vi "sensitivity.vi"(9 "x":dbl, 11 "sensitivity":dbl) -> (3 "scaled value":dbl)   [LabVIEW 2018]
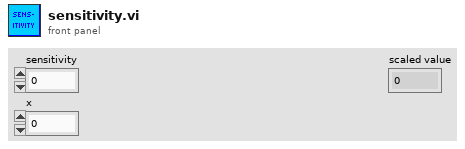
[diagram p1: front panel]
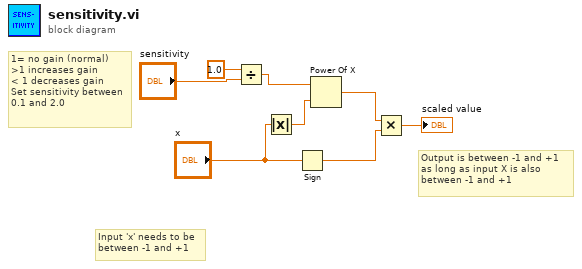
[diagram p0: block diagram]
diagram:
  # "Input 'x' needs to be\nbetween -1 and +1"
  # "Output is between -1 and +1\nas long as input X is also\nbetween -1 and +1"
  # "1= no gain (normal)\n>1 increases gain\n< 1 decreases gain\nSet sensitivity between\n0.1 and 2.0"
  n1 = Divide(x=1.0, y="sensitivity") -> (x/y=w8:dbl)
  n2 = Absolute Value(x="x") -> (abs(x)=w5:dbl)
  n3 = Sign(1:"x") -> (0:w2:dbl)
  n4 = Power Of X(1:w5, 2:w8) -> (0:w3:dbl)
  n5 = Multiply(x=w3, y=w2) -> (x*y=→"scaled value":dbl)
